vi "Configure Reading Memory.vi"(8 "error in (no error)":errorcluster, 10 "Measurement Counts (1)":i32=1, 11 "VISA resource name":refnum<visa-resource-name>) -> (0 "error out":errorcluster, 3 "VISA resource name out":refnum<visa-resource-name>)   [LabVIEW 2020, in "Agilent 3446X Series.lvlib"]
doc: "Specifies the number of measurements to store in reading memory before setting bit 9 in the Standard Operation Register group event register to 1.\n\n<b>Note(s):</b>\nThis vi is not supported for EDU34450A model."
uses:
  Agilent 3446X Series.lvlib
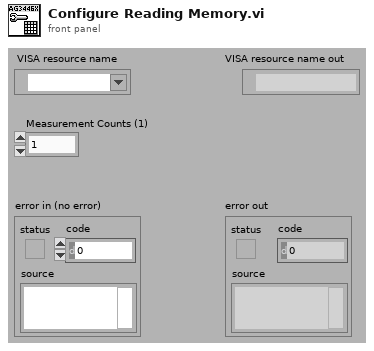
[diagram p1: front panel]
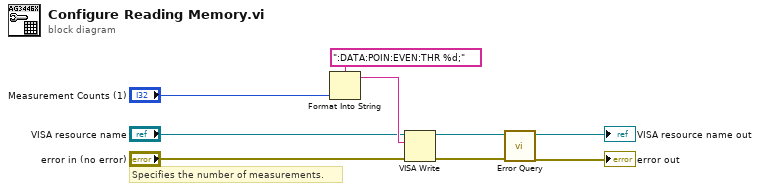
[diagram p0: block diagram]
diagram:
  # "Specifies the number of measurements."
  n1 = Format Into String(format string=":DATA:POIN:EVEN:THR %d;", "Measurement Counts (1)") -> (resulting string=w7:string)  [unwired: 2 in, 1 out]
  n2 = VISA Write(VISA resource name="VISA resource name", write buffer=w7, error in (no error)="error in (no error)") -> (VISA resource name out=w4:refnum<visa-resource-name>, error out=w3:errorcluster)  [unwired: 1 out]
  n3 = call "Error Query.vi"("error in (no error)"=w3, "VISA resource name"=w4) -> ("error out"=→"error out":errorcluster, "VISA resource name out"=→"VISA resource name out":refnum<visa-resource-name>)  [unwired: 8 out]
